vi "get desired keys.vi"(8 "error in":errorcluster, 11 "WaveformAcq configuration in":refnum<class "WaveformAcq configuration.lvclass">) -> (0 "error out":errorcluster, 2 "desired keys":string[](array[string]), 3 "WaveformAcq configuration out":refnum<class "WaveformAcq configuration.lvclass">)   [LabVIEW 2017, in "WaveformAcq configuration.lvclass"]
uses:
  WaveformAcq configuration.lvclass
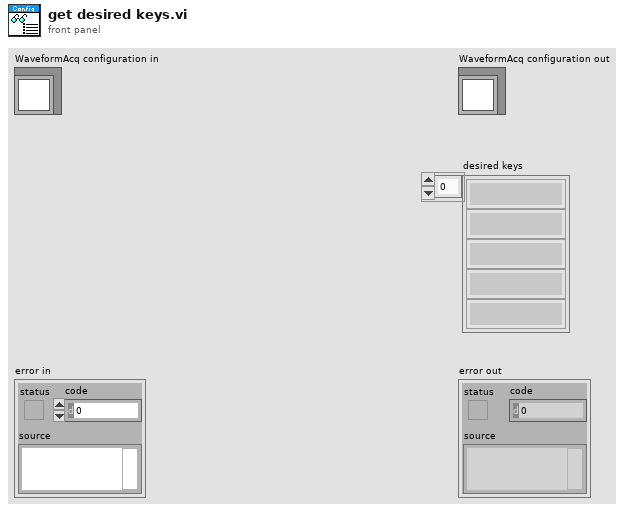
[diagram p1: front panel]
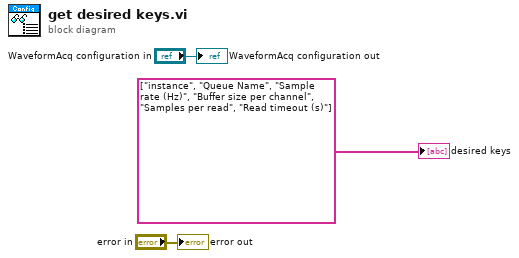
[diagram p0: block diagram]
diagram:
  "error out" <- "error in"
  "WaveformAcq configuration out" <- "WaveformAcq configuration in"
  "desired keys" <- string[] ["instance", "Queue Name", "Sample rate (Hz)", "Buffer size per channel", "Samples per read", "Read timeout (s)"] ("desired keys")
